vi "MQTT FGV net.vi"(6 "Options":T1, 7 "topics":string[](array[string]), 8 "error in (no error)":errorcluster, 10 "Message":string, 11 "Topic":string) -> (0 "error out":errorcluster, 1 "Error Info":string, 2 "messagereceived":string[](array[string]), 3 "topicrecieved":string[](array[string]), 5 "Connected":bool)   [LabVIEW 2017]
uses:
  Controls/MQTT FGV Options.ctl
  D:/Software Codes/Framework/Source Code/Auto Run Screen/Source Code/IPC/MQTT/Support/MQTTdll.dll
  MQTTdll.dll
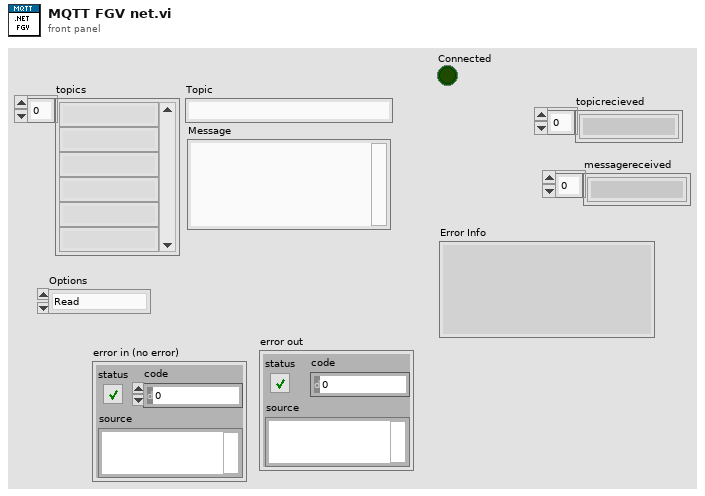
[diagram p1: front panel]
types:
  T1 = typedef "MQTT FGV Options.ctl" = enum16{"Read", "Subscribe", "Publish", "Get Status", "Connect", "Disconnect"}
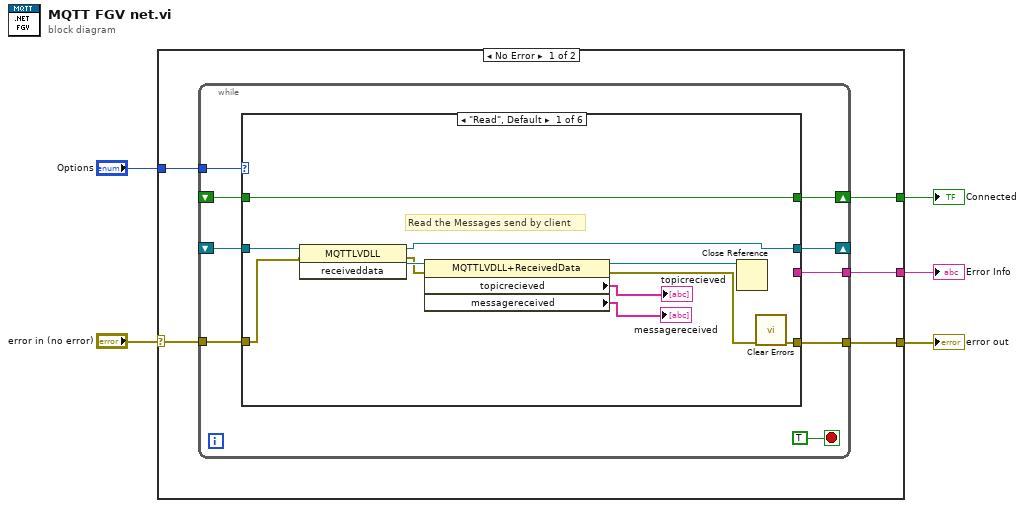
[diagram p0: block diagram]
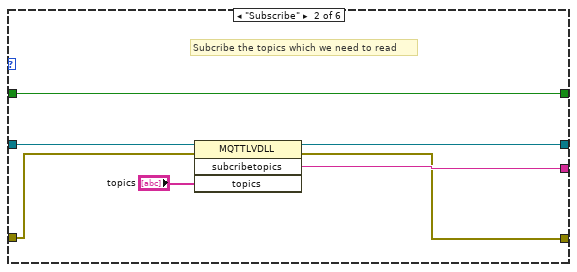
[diagram p2: hidden frame]
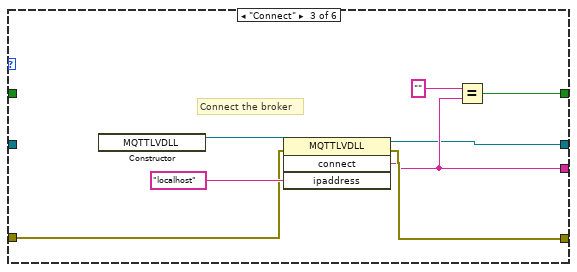
[diagram p3: hidden frame]
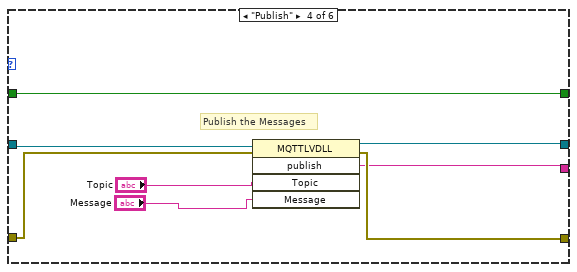
[diagram p4: hidden frame]
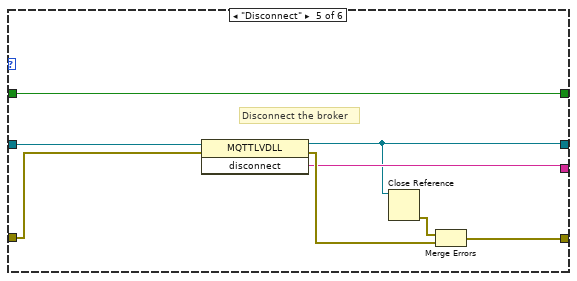
[diagram p5: hidden frame]
diagram:
  n1 = case shown="No Error" "error in (no error)" {
    selector: "error in (no error)" -> [w6 w65]
    tunnel: "Options" -> [w10 _]
    tunnel: [w9 _] -> w4
    tunnel: [w8 w65] -> w3
    tunnel: [w7 _] -> w2
    frame No Error {
      n2 = while {
        tunnel: w10 -> [w19]
        tunnel: [w17] -> w9
        tunnel: w6 -> [w16]
        tunnel: [w15] -> w8
        shift-right: [w14] -> w7
        shift-left: _ -> [w13]
        shift-right: [w12] -> _
        shift-left: _ -> [w11]
        stop <- TRUE stop-if-true
        n3 = case shown="\"Read\", Default" w19 {
          tunnel: [_ w32 w39 w46 w55 _] -> w17
          tunnel: w16 -> [w26 w33 w41 w49 w56 w63]
          tunnel: [w22 w31 w40 w50 w61 w63] -> w15
          tunnel: [w30 w37 w44 w53 w60 w64] -> w14
          tunnel: w13 -> [w30 w37 _ w53 w60 w64]
          tunnel: [w25 w35 w38 w51 w54 w62] -> w12
          tunnel: w11 -> [w29 w36 _ w52 w59 w62]
          frame "Read", Default {
            # "Read the Messages send by client"
            n4 = invoke class="MQTTLVDLL" method="receiveddata"(reference=w29, error in=w26) -> (reference out=w25:refnum<k24>, error out=w27:errorcluster, "receiveddata"=w28:refnum<k24>)  [unwired: 1 in]
            n5 = property class="MQTTLVDLL+ReceivedData"(reference=w28, error in=w27) -> (reference out=w23:refnum<k24>, error out=w24:errorcluster, "topicrecieved"=→"topicrecieved":string[], "messagereceived"=→"messagereceived":string[])
            n6 = Close Reference(reference=w23) -> ()  [unwired: 1 in, 1 out]
            n7 = call <vilib>:"Clear Errors.vi"("error in (no error)"=w24) -> ("error out"=w22:errorcluster)  [unwired: 5 in, 1 out]
          }
          frame "Subscribe" {
            # "Subcribe the topics which we need to read"
            n8 = invoke class="MQTTLVDLL" method="subcribetopics"(reference=w36, error in=w33, "topics"="topics") -> (reference out=w35:refnum<k24>, error out=w31:errorcluster, "subcribetopics"=w32:string)  [unwired: 1 in, 1 out]
          }
          frame "Connect" {
            # "Connect the broker"
            n9 = constructor class="MQTTLVDLL"() -> (reference out=w43:refnum<k24>)  [unwired: 3 in, 2 out]
            n10 = invoke class="MQTTLVDLL" method="connect"(reference=w43, error in=w41, "ipaddress"="localhost") -> (reference out=w38:refnum<k24>, error out=w40:errorcluster, "connect"=w39:string)  [unwired: 1 in, 1 out]
            n11 = Equal?(x="", y=w39) -> (x = y?=w44:bool)
          }
          frame "Publish" {
            # "Publish the Messages"
            n12 = invoke class="MQTTLVDLL" method="publish"(reference=w52, error in=w49, "Topic"="Topic", "Message"="Message") -> (reference out=w51:refnum<k24>, error out=w50:errorcluster, "publish"=w46:string)  [unwired: 1 in, 2 out]
          }
          frame "Disconnect" {
            # "Disconnect the broker"
            n13 = invoke class="MQTTLVDLL" method="disconnect"(reference=w59, error in=w56) -> (reference out=w54:refnum<k24>, error out=w57:errorcluster, "disconnect"=w55:string)  [unwired: 1 in]
            n14 = Close Reference(reference=w54) -> (error out=w58:errorcluster)  [unwired: 1 in]
            n15 = Merge Errors(w58, w57) -> (w61:errorcluster)
          }
          frame "Get Status" {
            # "Get the Connection Status"
          }
        }
      }
    }
    frame Error {
      # "Error"
    }
  }
  "Error Info" <- w4
  "error out" <- w3
  "Connected" <- w2
